vi "populateListbox.vi"(8 "error in (no error)":errorcluster, 11 "BaseSetting in":refnum<class "Setting.lvclass">) -> (0 "error out":errorcluster, 3 "BaseSetting out":refnum<class "Setting.lvclass">)   [LabVIEW 2016, in "Settings.lvlib" / "Setting.lvclass"]
uses:
  Setting.lvclass
  Setting.lvclass/Setting.ctl
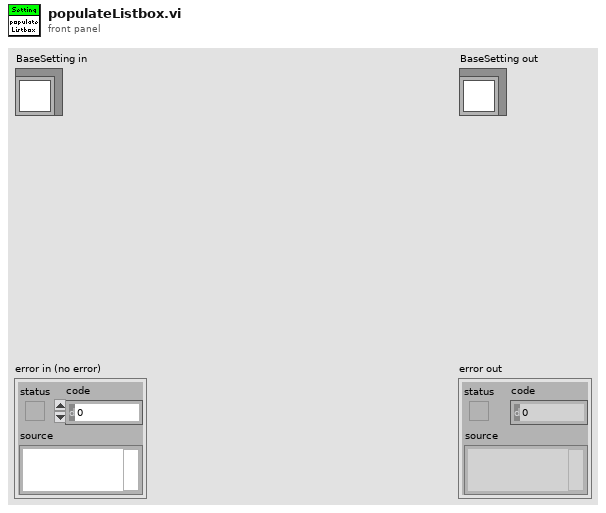
[diagram p1: front panel]
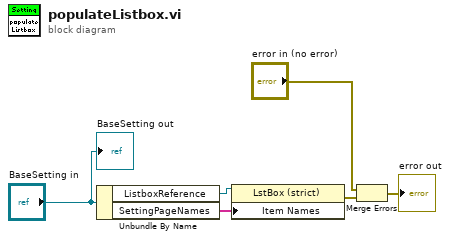
[diagram p0: block diagram]
diagram:
  n1 = Unbundle By Name("BaseSetting in") -> ("ListboxReference"=w5:refnum<vi>, "SettingPageNames"=w4:string[])
  n2 = property on="Property Node" class="LstBox (strict)"(reference=w5, "Item Names"=w4) -> (error out=w2:errorcluster)  [unwired: 1 in, 1 out]
  n3 = Merge Errors("error in (no error)", w2) -> (→"error out":errorcluster)
  "BaseSetting out" <- "BaseSetting in"
